vi "ConfigureSetpoints.vi"(6 "Apply New Setpoint":bool, 8 "New Setpoint":dbl, 9 "Selected Setpoint Index":i32, 10 "Setpoint Save Location":path, 11 "Setpoint Names":string[](array[string])) -> (0 "Selected Setpoint Value":dbl, 3 "Setpoints":dbl[](array[numeric]))   [LabVIEW 2019]
doc: "This VI allows the user to change setpoints from the FRC 4265 dashboard and save them to the roboRIO."
uses:
  <vilib>/Utility/xml.llb/Write to XML File(string).vi
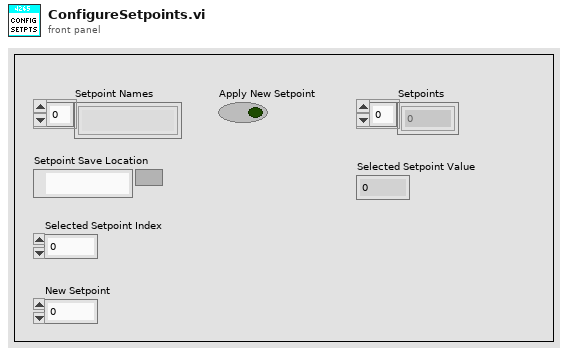
[diagram p1: front panel]
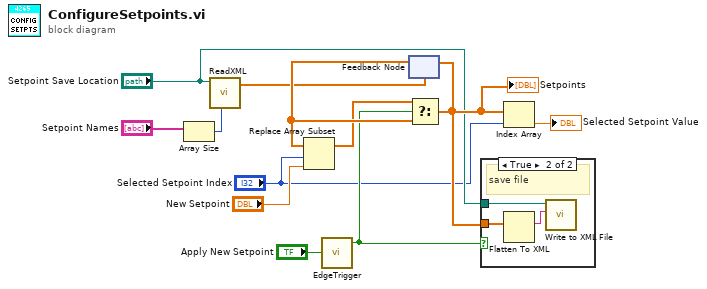
[diagram p0: block diagram]
diagram:
  n1 = Array Size(array="Setpoint Names") -> (size(s)=w3:i32)
  n2 = call "ReadXML.vi"("Default Number of Elements"=w3, "File Path (.xml)"="Setpoint Save Location") -> ("Data"=w4:dbl[])  [unwired: 8 in, 1 out]
  n3 = call "EdgeTrigger.vi"("Input Signal"="Apply New Setpoint") -> ("Rising Edge Trigger"=w8:bool)  [unwired: 2 out]
  n4 = feedback #1(w4) -> (w12:dbl[])
  n5 = Replace Array Subset(array=w12, new element="New Setpoint", index="Selected Setpoint Index") -> (w5:dbl[])
  n6 = Select(t=w5, s=w8, f=w12) -> (s? t:f=w10:dbl[])
  "Setpoints" <- w10
  n7 = feedback-in #1(w10) -> ()
  n8 = case shown="True" w8 {
    tunnel: w10 -> [_ w14]
    tunnel: "Setpoint Save Location" -> [_ w13]
    frame False {
    }
    frame True {
      # "save file"
      n9 = Flatten To XML(anything=w14) -> (xml string=w15:string)
      n10 = call-poly <vilib>:"Write to XML File.vi"("XML Input"=w15, "XML File Path"=w13) -> ()  [unwired: 7 in, 3 out]
    }
  }
  n11 = Index Array(array=w10, index="Selected Setpoint Index") -> (element=→"Selected Setpoint Value":dbl)
